vi "CH1_Comm_TCPIP_NEW.vi"() -> ()   [LabVIEW 2018]
uses:
  RxTx/CCS_RxTx.lvclass
panel:
  in  "stop":bool
  in  "IP 2":string="200.131.64.49"
  out "error out 5":errorcluster
  out "error out 4":errorcluster
  out "error out 3":errorcluster
  out "error out 2":errorcluster
  in  "RxTx.lvclass 2":refnum<class "CCS_RxTx.lvclass">
  in  "Channel":u16=1
  # "Channel 1 - TCPIP Communication"
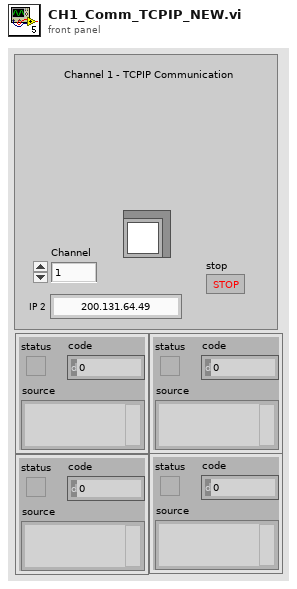
[diagram p1: front panel]
types:
  T1 = enum16{"Standard", "Buffered", "CRLF", "Immediate"}
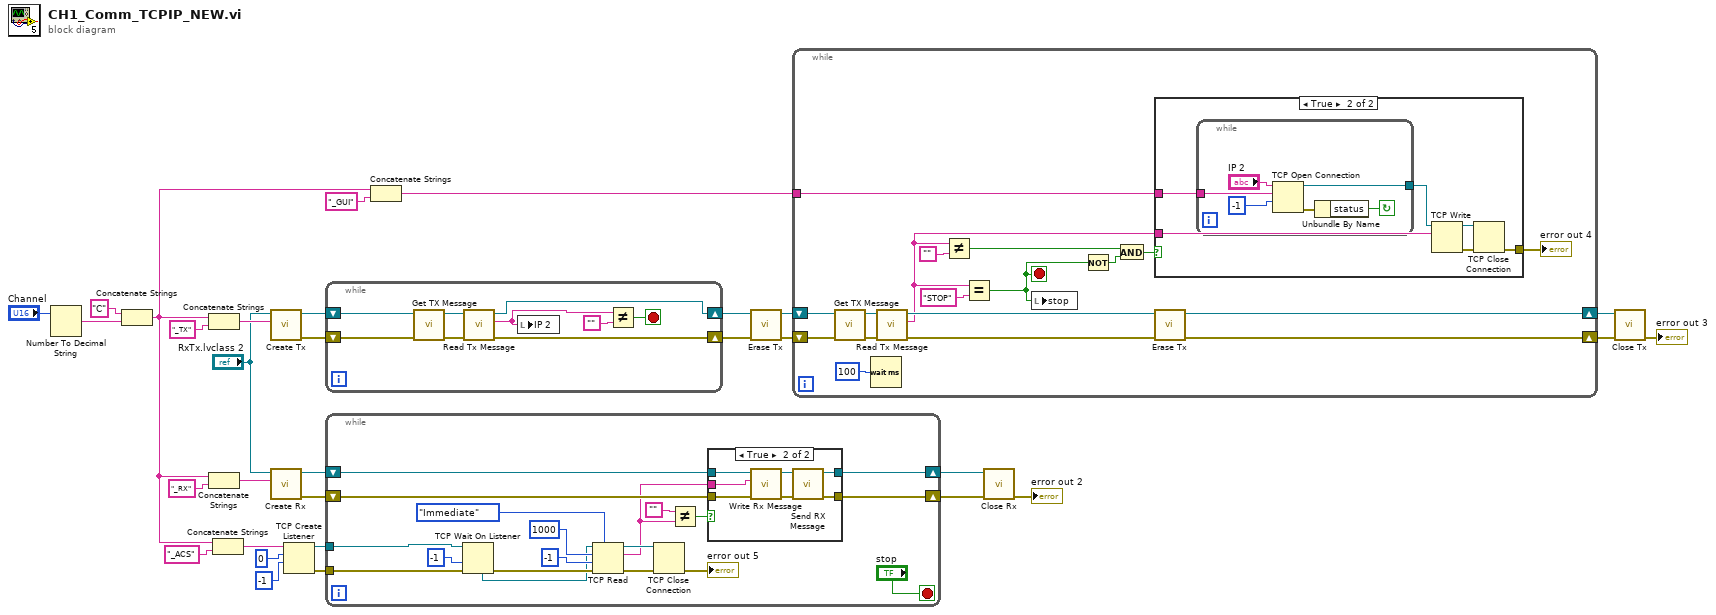
[diagram p0: block diagram]
diagram:
  n1 = Number To Decimal String(number="Channel") -> (decimal integer string=w28:string)  [unwired: 1 in]
  n2 = Concatenate Strings("C", w28) -> (w10:string)
  n3 = Concatenate Strings(w10, "_TX" ("Reader Name")) -> (w24:string)
  n4 = Concatenate Strings(w10, "_RX" ("Reader Name")) -> (w31:string)
  n5 = Concatenate Strings(w10, "_ACS" ("Reader Name")) -> (w15:string)
  n6 = call "Create Tx.vi"("Writer Name"=w24, "RxTx in"="RxTx.lvclass 2") -> ("error out"=w8:errorcluster, "RxTx out"=w9:refnum<class "CCS_RxTx.lvclass">)  [unwired: 8 in]
  n7 = call "Create Rx.vi"("Reader Name"=w31, "RxTx in"="RxTx.lvclass 2") -> ("error out"=w26:errorcluster, "RxTx out"=w27:refnum<class "CCS_RxTx.lvclass">)  [unwired: 8 in]
  n8 = TCP Create Listener(9:-1 ("timeout ms (25000)"), 10:u16 0 ("port"), 11:w15) -> (0:w12:errorcluster, 3:w13:refnum<k5>)  [unwired: 2 in, 1 out]
  n9 = while {
    shift-right: [w38] -> w7
    shift-left: w9 -> [w40]
    shift-right: [w37] -> w5
    shift-left: w8 -> [w35]
    stop <- w33 stop-if-true
    n10 = call "Get TX Message.vi"("error in (no error)"=w35, "RxTx in"=w40) -> ("error out"=w36:errorcluster, "RxTx out"=w39:refnum<class "CCS_RxTx.lvclass">)  [unwired: 8 in]
    n11 = call "Read Tx Message.vi"("error in (no error)"=w36, "RxTx in"=w39) -> ("error out"=w37:errorcluster, "Tx Message"=w32:string, "RxTx out"=w38:refnum<class "CCS_RxTx.lvclass">)  [unwired: 7 in]
    n12 = local write "IP 2"(w32) -> ()
    n13 = Not Equal?(x=w32, y="") -> (x != y?=w33:bool)
  }
  n14 = while {
    shift-right: [w42] -> w1
    shift-left: w26 -> [w59]
    shift-right: [w55] -> w3
    shift-left: w27 -> [w58]
    tunnel: w13 -> [w54]
    tunnel: w12 -> [w45]
    stop <- "stop" stop-if-true
    n15 = TCP Wait On Listener(8:w45, 9:-1 ("timeout ms (wait forever: -1)"), 11:w54) -> (0:w49:errorcluster, 4:w44:refnum<k5>)  [unwired: 1 in, 3 out]
    n16 = TCP Read(connection ID=w44, bytes to read=1000, error in (no error)=w49, 7:T1."Immediate" ("mode (standard)"), 9:-1 ("timeout ms (25000)")) -> (connection ID out=w47:refnum<k5>, data out=w43:string, error out=w46:errorcluster)
    n17 = TCP Close Connection(connection ID=w47, error in (no error)=w46) -> (error out=→"error out 5":errorcluster)  [unwired: 1 in, 1 out]
    n18 = Not Equal?(x="", y=w43) -> (x != y?=w56:bool)
    n19 = case shown="True" w56 {
      tunnel: w59 -> [w60 w66]
      tunnel: w58 -> [w61 w65]
      tunnel: [w61 w64] -> w55
      tunnel: [w60 w63] -> w42
      tunnel: w43 -> [_ w62]
      frame False {
      }
      frame True {
        n20 = call "Write Rx Message.vi"("error in (no error)"=w66, "Rx Message"=w62, "RxTx in"=w65) -> ("error out"=w67:errorcluster, "RxTx out"=w68:refnum<class "CCS_RxTx.lvclass">)  [unwired: 7 in]
        n21 = call "Send RX Message.vi"("error in (no error)"=w67, "RxTx in"=w68) -> ("error out"=w63:errorcluster, "RxTx out"=w64:refnum<class "CCS_RxTx.lvclass">)  [unwired: 8 in]
      }
    }
  }
  n22 = Concatenate Strings(w10, "_GUI" ("Reader Name")) -> (w16:string)
  n23 = call "Erase Tx.vi"("error in (no error)"=w5, "RxTx in"=w7) -> ("error out"=w2:errorcluster, "RxTx out"=w6:refnum<class "CCS_RxTx.lvclass">)  [unwired: 8 in]
  n24 = while {
    shift-right: [w86] -> w22
    shift-left: w6 -> [w80]
    shift-right: [w75] -> w4
    shift-left: w2 -> [w79]
    tunnel: w16 -> [w76]
    stop <- w70 stop-if-true
    n25 = call "Get TX Message.vi"("error in (no error)"=w79, "RxTx in"=w80) -> ("error out"=w85:errorcluster, "RxTx out"=w81:refnum<class "CCS_RxTx.lvclass">)  [unwired: 8 in]
    n26 = Wait (ms)(milliseconds to wait=u32 100) -> ()  [unwired: 1 out]
    n27 = call "Read Tx Message.vi"("error in (no error)"=w85, "RxTx in"=w81) -> ("error out"=w82:errorcluster, "Tx Message"=w74:string, "RxTx out"=w83:refnum<class "CCS_RxTx.lvclass">)  [unwired: 7 in]
    n28 = Not Equal?(x=w74, y="") -> (x != y?=w72:bool)
    n29 = Equal?(x=w74, y="STOP") -> (x = y?=w70:bool)
    n30 = local write "stop"(w70) -> ()
    n31 = Not(x=w70) -> (.not. x?=w69:bool)
    n32 = And(x=w72, y=w69) -> (x .and. y?=w71:bool)
    n33 = case shown="True" w71 {
      tunnel: w74 -> [_ w91]
      tunnel: [_ w87] -> w78
      tunnel: w76 -> [_ w92]
      frame False {
      }
      frame True {
        n34 = while {
          tunnel: w92 -> [w97]
          tunnel: [w94] -> w90
          stop <- w98 continue-if-true
          n35 = TCP Open Connection(address="IP 2", remote port or service name=w97, timeout ms (60000)=-1 ("timeout")) -> (connection ID=w94:refnum<k5>, error out=w96:errorcluster)  [unwired: 2 in]
          n36 = Unbundle By Name(w96) -> ("status"=w98:bool)
        }
        n37 = TCP Write(connection ID=w90, data in=w91) -> (connection ID out=w88:refnum<k5>, error out=w89:errorcluster)  [unwired: 2 in, 1 out]
        n38 = TCP Close Connection(connection ID=w88, error in (no error)=w89) -> (error out=w87:errorcluster)  [unwired: 1 in, 1 out]
      }
    }
    "error out 4" <- w78
    n39 = call "Erase Tx.vi"("error in (no error)"=w82, "RxTx in"=w83) -> ("error out"=w75:errorcluster, "RxTx out"=w86:refnum<class "CCS_RxTx.lvclass">)  [unwired: 8 in]
  }
  n40 = call "Close Rx.vi"("error in (no error)"=w1, "RxTx in"=w3) -> ("error out"=→"error out 2":errorcluster)  [unwired: 8 in, 1 out]
  n41 = call "Close Tx.vi"("error in (no error)"=w4, "RxTx in"=w22) -> ("error out"=→"error out 3":errorcluster)  [unwired: 8 in, 1 out]
